vi "Fully Dynamic FPGA Interface Example.vi"() -> ()   [LabVIEW 2011]
uses:
  TypeDefs/Fully Dynamic FPGA Interface TypeDef.ctl
  <vilib>/Utility/sysdir.llb/System Directory Type.ctl
  <userlib>/_FPGA Interface Advanced Tools/FPGA Interface Base/FPGA Interface Base.lvclass
  <userlib>/_FPGA Interface Advanced Tools/FPGA Bitfile Utility/Get Register Map.vi
  <userlib>/_FPGA Interface Advanced Tools/FPGA Bitfile Utility/Get Base Address.vi
  <vilib>/rvi/Utilities/XML/nirviXML_GetValue.vi
  <vilib>/rvi/Utilities/XML/nirviXML_GetValue_String.vi
  <vilib>/rvi/Bitfile/niFpgaReadBitfileXml_VIRegisterMap.vi
  <vilib>/rvi/Utilities/XML/nirviXML_GetValue_U32.vi
  <vilib>/Utility/VariantDataType/GetTypeInfo.vi
  <vilib>/Utility/VariantDataType/GetArrayInfo.vi
  <userlib>/_FPGA Interface Advanced Tools/FPGA Interface Base/FPGA Read By Name - Boolean.vi
  <userlib>/_FPGA Interface Advanced Tools/FPGA Interface Base/FPGA Read By Name - I8.vi
  <userlib>/_FPGA Interface Advanced Tools/FPGA Interface Base/FPGA Read By Name - I16.vi
  <userlib>/_FPGA Interface Advanced Tools/FPGA Interface Base/FPGA Read By Name - I32.vi
  <userlib>/_FPGA Interface Advanced Tools/FPGA Interface Base/FPGA Read By Name - I64.vi
  <userlib>/_FPGA Interface Advanced Tools/FPGA Interface Base/FPGA Read By Name - U8.vi
  <userlib>/_FPGA Interface Advanced Tools/FPGA Interface Base/FPGA Read By Name - U16.vi
  <userlib>/_FPGA Interface Advanced Tools/FPGA Interface Base/FPGA Read By Name - U32.vi
  <userlib>/_FPGA Interface Advanced Tools/FPGA Interface Base/FPGA Read By Name - U64.vi
  <userlib>/_FPGA Interface Advanced Tools/FPGA Interface Base/FPGA Read Array By Name - Boolean.vi
  <userlib>/_FPGA Interface Advanced Tools/FPGA Interface Base/FPGA Read Array By Name - I8.vi
  <userlib>/_FPGA Interface Advanced Tools/FPGA Interface Base/FPGA Read Array By Name - I16.vi
  <userlib>/_FPGA Interface Advanced Tools/FPGA Interface Base/FPGA Read Array By Name - I32.vi
  <userlib>/_FPGA Interface Advanced Tools/FPGA Interface Base/FPGA Read Array By Name - I64.vi
  <userlib>/_FPGA Interface Advanced Tools/FPGA Interface Base/FPGA Read Array By Name - U8.vi
  <userlib>/_FPGA Interface Advanced Tools/FPGA Interface Base/FPGA Read Array By Name - U16.vi
  <userlib>/_FPGA Interface Advanced Tools/FPGA Interface Base/FPGA Read Array By Name - U32.vi
  <userlib>/_FPGA Interface Advanced Tools/FPGA Interface Base/FPGA Read Array By Name - U64.vi
  <userlib>/_FPGA Interface Advanced Tools/FPGA Interface Base/FPGA Write By Name - Boolean.vi
  <userlib>/_FPGA Interface Advanced Tools/FPGA Interface Base/FPGA Write By Name - I8.vi
  <userlib>/_FPGA Interface Advanced Tools/FPGA Interface Base/FPGA Write By Name - I16.vi
  <userlib>/_FPGA Interface Advanced Tools/FPGA Interface Base/FPGA Write By Name - I32.vi
  <userlib>/_FPGA Interface Advanced Tools/FPGA Interface Base/FPGA Write By Name - I64.vi
  <userlib>/_FPGA Interface Advanced Tools/FPGA Interface Base/FPGA Write By Name - U8.vi
  <userlib>/_FPGA Interface Advanced Tools/FPGA Interface Base/FPGA Write By Name - U16.vi
  <userlib>/_FPGA Interface Advanced Tools/FPGA Interface Base/FPGA Write By Name - U32.vi
  <userlib>/_FPGA Interface Advanced Tools/FPGA Interface Base/FPGA Write By Name - U64.vi
  <userlib>/_FPGA Interface Advanced Tools/FPGA Interface Base/FPGA Write Array By Name - Boolean.vi
  <userlib>/_FPGA Interface Advanced Tools/FPGA Interface Base/FPGA Write Array By Name - I8.vi
  <userlib>/_FPGA Interface Advanced Tools/FPGA Interface Base/FPGA Write Array By Name - I16.vi
  <userlib>/_FPGA Interface Advanced Tools/FPGA Interface Base/FPGA Write Array By Name - I32.vi
  <userlib>/_FPGA Interface Advanced Tools/FPGA Interface Base/FPGA Write Array By Name - I64.vi
  <userlib>/_FPGA Interface Advanced Tools/FPGA Interface Base/FPGA Write Array By Name - U8.vi
  <userlib>/_FPGA Interface Advanced Tools/FPGA Interface Base/FPGA Write Array By Name - U16.vi
  <userlib>/_FPGA Interface Advanced Tools/FPGA Interface Base/FPGA Write Array By Name - U32.vi
  <userlib>/_FPGA Interface Advanced Tools/FPGA Interface Base/FPGA Write Array By Name - U64.vi
  <userlib>/_FPGA Interface Advanced Tools/FPGA Bitfile Utility/FPGA Bitfile Utility.lvlib
panel:
  in  "RIO Resource":refnum<visa-resource-name>="RIO0"
  out "Boolean Array Read":bool[](array[boolean])
  in  "Boolean Array Write":bool[](array[boolean])
  in  "Numeric Array Write":dbl[](array[numeric])
  out "Numeric Array Read":dbl[](array[numeric])
  in  "Numeric Write":dbl
  out "Numeric Read":dbl
  in  "Boolean Write":bool
  out "Bool Read":bool
  in  "Write":bool
  in  "Read":bool
  in  "Multicolumn Listbox":i32(listbox)
  in  "Stop FPGA":bool
  in  "Run FPGA":bool
  in  "Select Bitfile":bool
  out "Bifile Path":path
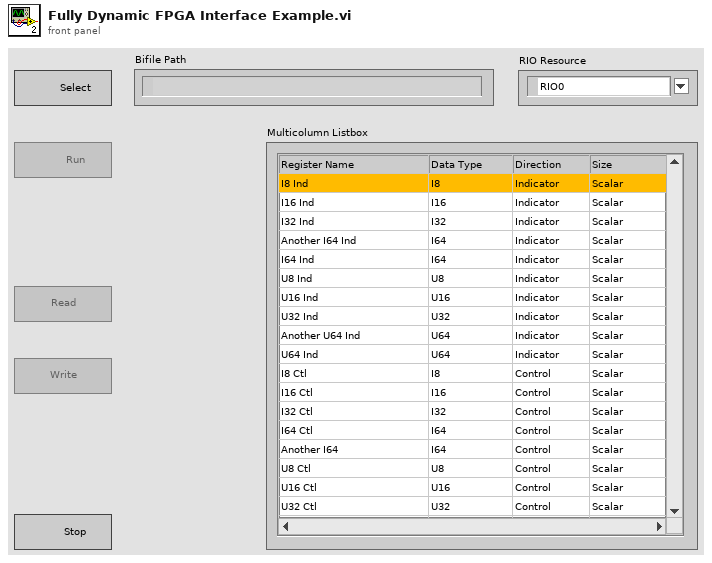
[diagram p1: front panel]
types:
  T1 = typedef "Fully Dynamic FPGA Interface TypeDef.ctl" = enum16{"Idle", "Init", "Read", "Write"}
  T2 = enum8{"Enabled", "Disabled", "Disabled and Grayed Out"}
  T3 = typedef "System Directory Type.ctl" = i32
  T4 = typedef "FPGA Bitfile Utility.lvlib/Control_Indicator Info.ctl" = cluster{"Array?":bool, "Data Type":T5, "Address":u32, "Num Elements":u32, "Name":string}
  T5 = typedef "niFpgaDataTypeControl.ctl" = enum32{"Boolean", "I8", "I16", "I32", "I64", "U8", "U16", "U32", "U64", "FXP", "CustomControl"}
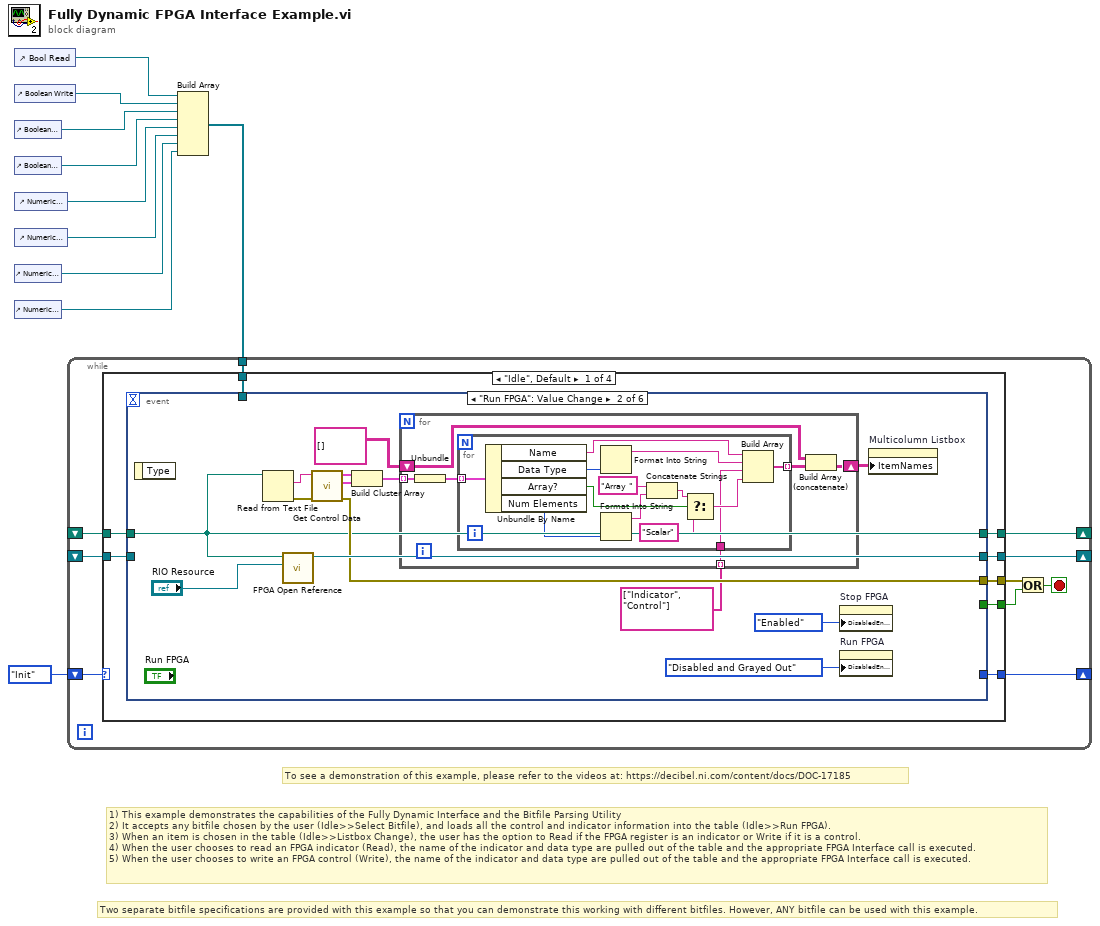
[diagram p0: block diagram]
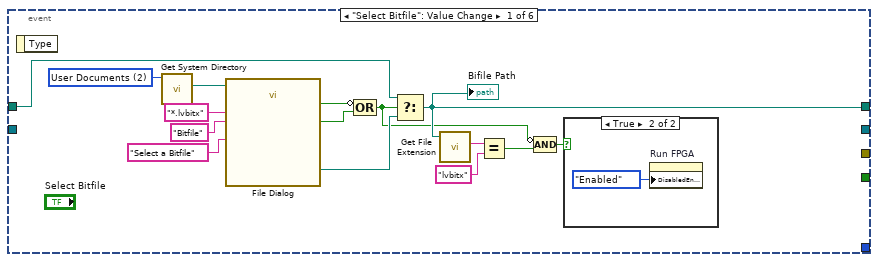
[diagram p2: hidden frame]
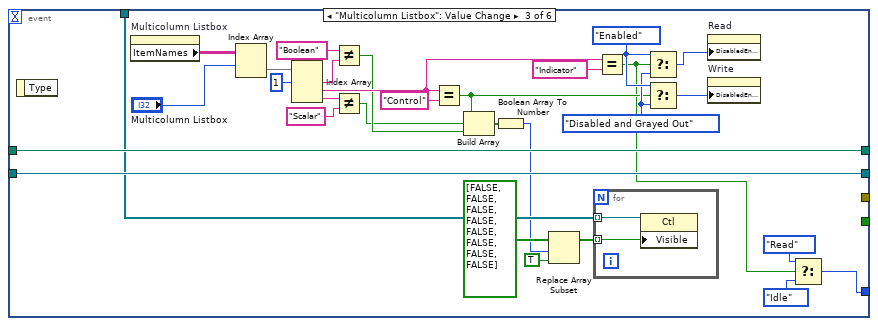
[diagram p4: hidden frame]
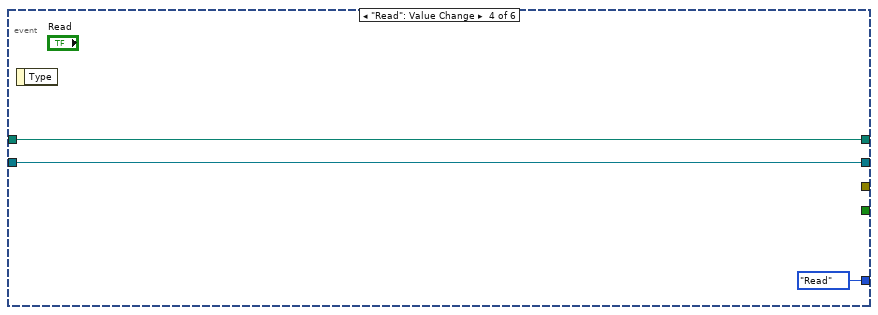
[diagram p5: hidden frame]
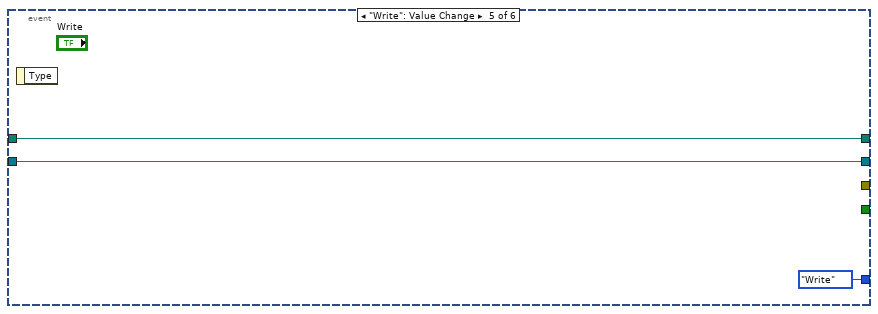
[diagram p6: hidden frame]
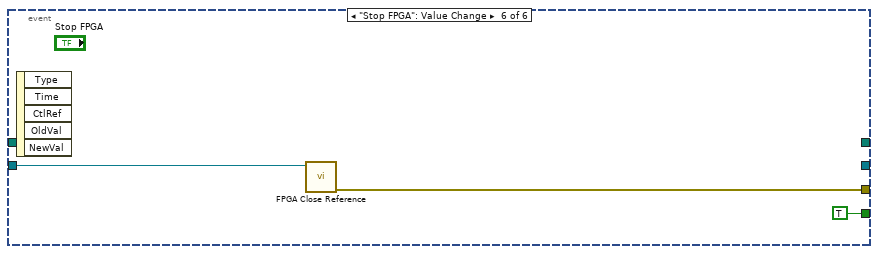
[diagram p7: hidden frame]
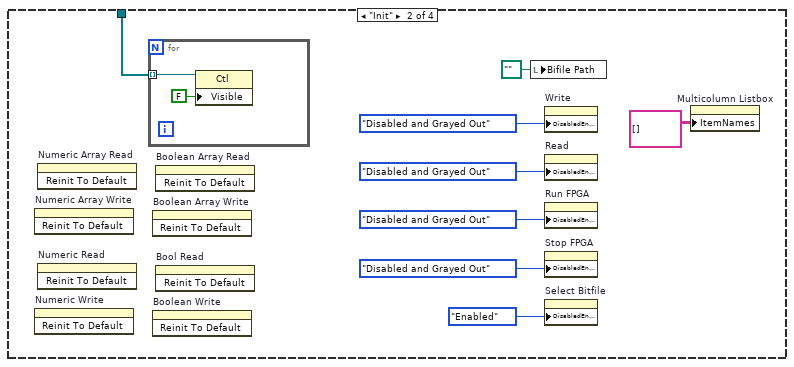
[diagram p8: hidden frame]
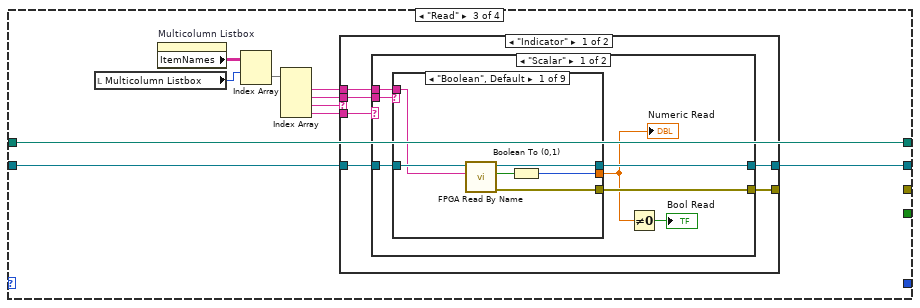
[diagram p9: hidden frame]
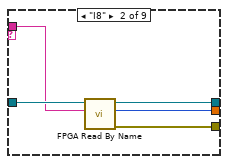
[diagram p10: hidden frame]
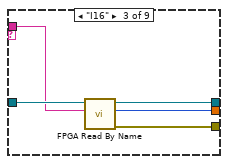
[diagram p11: hidden frame]
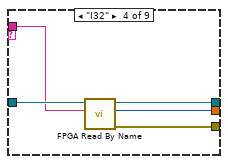
[diagram p12: hidden frame]
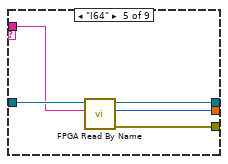
[diagram p13: hidden frame]
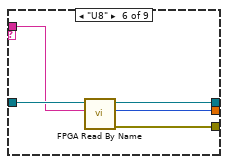
[diagram p14: hidden frame]
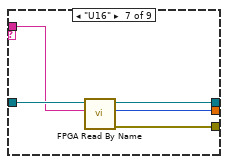
[diagram p15: hidden frame]
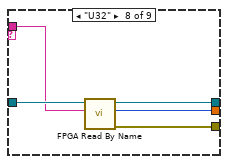
[diagram p16: hidden frame]
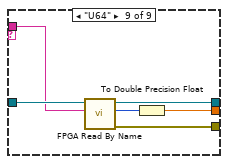
[diagram p17: hidden frame]
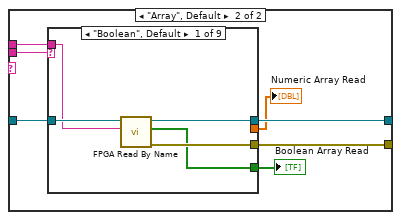
[diagram p18: hidden frame]
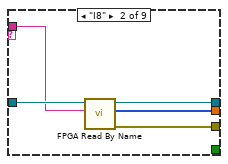
[diagram p19: hidden frame]
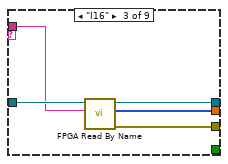
[diagram p20: hidden frame]
diagram:
  # "Two separate bitfile specifications are provided with this example so that you can demonstrate this working with different bitfiles. However, ANY bitfile can be used with this example."
  # "1) This example demonstrates the capabilities of the Fully Dynamic Interface and the Bitfile Parsing Utility\n2) It accepts any bitfile chosen by the user (Idle>>Select Bitfile), and loads all the control and indicator information into the table (Idle>>Run FPGA).\n3) When an item is chosen in the table (Idle>>Listbox Change), the user has the option to Read if the FPGA register is an indicator or Write if it is a control.\n4) When the user chooses to read an FPGA indicator (Read), the name of the indicator and data type are pulled out of the table and the appropriate FPGA Interface call is executed.\n5) When the user chooses to write an FPGA control (Write), the name of the indicator and data type are pulled out of the table and the appropriate FPGA Interface call is executed."
  # "To see a demonstration of this example, please refer to the videos at: https://decibel.ni.com/content/docs/DOC-17185"
  n1 = control-ref of="Bool Read"() -> (w10:refnum<vi>)
  n2 = control-ref of="Boolean Write"() -> (w6:refnum<vi>)
  n3 = control-ref of="Boolean Array Read"() -> (w7:refnum<vi>)
  n4 = control-ref of="Boolean Array Write"() -> (w8:refnum<vi>)
  n5 = control-ref of="Numeric Read"() -> (w5:refnum<vi>)
  n6 = control-ref of="Numeric Write"() -> (w4:refnum<vi>)
  n7 = control-ref of="Numeric Array Read"() -> (w3:refnum<vi>)
  n8 = control-ref of="Numeric Array Write"() -> (w2:refnum<vi>)
  n9 = Build Array(w10, w6, w7, w8, w5, w4, w3, w2) -> (w9:refnum<vi>[])
  n10 = while {
    shift-right: [w20] -> _
    shift-left: _ -> [w19]
    shift-right: [w18] -> _
    shift-left: _ -> [w17]
    tunnel: w9 -> [w13]
    shift-right: [w11] -> _
    shift-left: Fully_Dynamic_FPGA_Interface_TypeDef."Init" -> [w12]
    stop <- w15 stop-if-true
    n11 = case shown="\"Idle\", Default" w12 {
      tunnel: [w28 _ w129 w253] -> w20
      tunnel: w19 -> [w27 _ w129 w253]
      tunnel: [w26 _ w130 w254] -> w18
      tunnel: w17 -> [w25 _ w131 w255]
      tunnel: [w24 _ _ _] -> w16
      tunnel: [w23 _ _ _] -> w14
      tunnel: w13 -> [w22 w119 _ _]
      tunnel: [w21 _ _ _] -> w11
      frame "Idle", Default {
        n12 = event shown="[1] \"Run FPGA\": Value Change" {
          selector: _ -> [_ _ _ _ _ _]
          dyn-events: _ -> [_ _ _ _ _ _]
          timeout: _ -> [_ _ _ _ _ _]
          tunnel: [w34 w54 w98 w111 w113 _] -> w28
          tunnel: w27 -> [w35 w54 w98 w111 w113 _]
          tunnel: [_ w58 w99 w110 w114 _] -> w26
          tunnel: w25 -> [_ _ w99 w110 w114 w118]
          tunnel: [_ w55 _ _ _ w117] -> w24
          tunnel: [_ _ _ _ _ TRUE] -> w23
          tunnel: w22 -> [_ _ w95 _ _ _]
          tunnel: [_ _ w80 Fully_Dynamic_FPGA_Interface_TypeDef."Read" Fully_Dynamic_FPGA_Interface_TypeDef."Write" _] -> w21
          event "Select Bitfile": Value Change {
            w43 = T3 2 items=["User Home"=0, "User Desktop"=1, "User Documents"=2, "User Application Data"=3, "User Preferences"=4, "User Temporary"=5, "Public Documents"=6, "Public Application Data"=7, "Public Preferences"=8, "Public Cache"=13, "System Core Libraries"=9, "System Installed Libraries"=10, "Application Files"=11, "Boot Volume Root"=12] ("system directory type")
            n13 = event-data() -> ()  [unwired: 1 in, 1 out]
            n14 = call <vilib>:"Get System Directory.vi"("system directory type"=w43) -> ("system directory"=w42:path)  [unwired: 10 in]
            n15 = call "File Dialog"("start path"=w42, "prompt"="Select a Bitfile", "pattern (all files)"="*.lvbitx", "pattern label"="Bitfile") -> ("selected path"=w36:path, "exists"=w37:bool, "cancelled"=w38:bool)  [unwired: 8 in, 1 out]
            n16 = Compound Arithmetic op=OR(invert w37, w38) -> (w29:bool)
            n17 = Select(t=w35, s=w29, f=w36) -> (s? t:f=w34:path)
            "Bifile Path" <- w34
            n18 = call <vilib>:"Get File Extension.vi"("file"=w34) -> ("lowercase file extension"=w33:string)  [unwired: 7 in, 3 out]
            n19 = Equal?(x=w33, y="lvbitx") -> (x = y?=w31:bool)
            n20 = Compound Arithmetic op=AND(invert w29, w31) -> (w30:bool)
            n21 = case shown="True" w30 {
              frame False {
              }
              frame True {
                n22 = property on="Run FPGA" class="Bool"("DisabledEnum"=T2."Enabled" ("Disabled")) -> ()  [unwired: 2 in, 2 out]
              }
            }
          }
          event "Run FPGA": Value Change {
            n23 = event-data() -> ()  [unwired: 1 in, 1 out]
            n24 = Read from Text File(file (use dialog)=w54) -> (text=w57:string, error out=w56:errorcluster)  [unwired: 3 in, 2 out]
            n25 = call <userlib>:"FPGA Open Reference.vi"("FPGA Resource"="RIO Resource", "Bitfile Path"=w54) -> ("FPGA Session"=w58:refnum<class "FPGA Interface Base.lvclass">)  [unwired: 8 in, 1 out]
            n26 = call <userlib>:"Get Control Data.vi"("error in (no error)"=w56, "bitfile xml in"=w57) -> ("error out"=w55:errorcluster, "Controls"=w51:T4[], "Indicators"=w53:T4[])  [unwired: 6 in, 1 out]
            n27 = Build Cluster Array(w53, w51) -> (w52:cluster{"Controls":T4[]}[])
            n28 = for {
              tunnel: w52 -> [w64] mode=indexing
              tunnel: string[] ["Indicator", "Control"] -> [w63] mode=indexing
              shift-right: [w62] -> w49
              shift-left: string[][] [] -> [w61]
              n29 = Unbundle(w64) -> ("Controls"=w59:T4[])
              n30 = for {
                tunnel: w59 -> [w77] mode=indexing
                tunnel: [w66] -> w60 mode=indexing
                tunnel: w63 -> [w65]
                n31 = Unbundle By Name(w77) -> ("Name"=w69:string, "Data Type"=w76:T5, "Array?"=w75:bool, "Num Elements"=w74:u32)
                n32 = Format Into String(w76) -> (resulting string=w68:string)  [unwired: 3 in, 1 out]
                n33 = Format Into String(w74) -> (resulting string=w72:string)  [unwired: 3 in, 1 out]
                n34 = Concatenate Strings("Array " ("Name"), w72) -> (w71:string)
                n35 = Select(t=w71, s=w75, f="Scalar" ("Name")) -> (s? t:f=w67:string)
                n36 = Build Array(w69, w68, w65, w67) -> (w66:string[])
              }
              n37 = Build Array (concatenate)(w61, w60) -> (w62:string[][])
            }
            n38 = property on="Stop FPGA" class="Bool"("DisabledEnum"=T2."Enabled" ("Disabled")) -> ()  [unwired: 2 in, 2 out]
            n39 = property on="Run FPGA" class="Bool"("DisabledEnum"=T2."Disabled and Grayed Out" ("Disabled")) -> ()  [unwired: 2 in, 2 out]
            n40 = property on="Multicolumn Listbox" class="MCListbox (strict)"("ItemNames"=w49) -> ()  [unwired: 2 in, 2 out]
          }
          event "Multicolumn Listbox": Value Change {
            w97 = T2."Disabled and Grayed Out" ("Disabled")
            w102 = T2."Enabled" ("Disabled")
            n41 = event-data() -> ()  [unwired: 1 in, 1 out]
            n42 = property on="Multicolumn Listbox" class="MCListbox (strict)"() -> ("ItemNames"=w107:string[][])  [unwired: 2 in, 2 out]
            n43 = Index Array(array=w107, index (row)="Multicolumn Listbox") -> (element=w103:string[])  [unwired: 1 in]
            n44 = Index Array(array=w103, index #1=1 ("index")) -> (element #1=w90:string, element #2=w91:string, element #3=w87:string)  [unwired: 2 in]
            n45 = Not Equal?(x="Boolean", y=w90) -> (x != y?=w88:bool)
            n46 = Not Equal?(x=w87, y="Scalar") -> (x != y?=w83:bool)
            n47 = Equal?(x=w91, y="Control") -> (x = y?=w79:bool)
            n48 = Build Array(w79, w83, w88) -> (w85:bool[])
            n49 = Boolean Array To Number(Boolean array=w85) -> (number=w84:u32)
            n50 = Replace Array Subset(array=bool[] [FALSE, FALSE, FALSE, FALSE, FALSE, FALSE, FALSE, FALSE], new element=TRUE ("new element/subarray"), index=w84) -> (w94:bool[])
            n51 = for {
              tunnel: w95 -> [w109] mode=indexing
              tunnel: w94 -> [w108] mode=indexing
              n52 = property class="Ctl"(reference=w109, "Visible"=w108) -> ()  [unwired: 1 in, 2 out]
            }
            n53 = Equal?(x=w91, y="Indicator") -> (x = y?=w78:bool)
            n54 = Select(t=w102, s=w78, f=w97) -> (s? t:f=w100:T2)
            n55 = Select(t=w102, s=w79, f=w97) -> (s? t:f=w101:T2)
            n56 = property on="Read" class="Bool"("DisabledEnum"=w100) -> ()  [unwired: 2 in, 2 out]
            n57 = property on="Write" class="Bool"("DisabledEnum"=w101) -> ()  [unwired: 2 in, 2 out]
            n58 = Select(t=Fully_Dynamic_FPGA_Interface_TypeDef."Read", s=w78, f=Fully_Dynamic_FPGA_Interface_TypeDef."Idle") -> (s? t:f=w80:T1)
          }
          event "Read": Value Change {
            n59 = event-data() -> ()  [unwired: 1 in, 1 out]
          }
          event "Write": Value Change {
            n60 = event-data() -> ()  [unwired: 1 in, 1 out]
          }
          event "Stop FPGA": Value Change {
            n61 = event-data() -> ()  [unwired: 1 in, 5 out]
            n62 = call-dynamic "FPGA Close Reference.vi"("FPGA Session In"=w118) -> ("error out"=w117:errorcluster)  [unwired: 10 in]
          }
        }
      }
      frame "Init" {
        n63 = invoke on="Numeric Array Write" class="Arr (strict)" method="Reinit To Default"() -> ()  [unwired: 3 in, 3 out]
        n64 = invoke on="Numeric Write" class="DigNum (strict)" method="Reinit To Default"() -> ()  [unwired: 3 in, 3 out]
        n65 = invoke on="Numeric Array Read" class="Arr (strict)" method="Reinit To Default"() -> ()  [unwired: 3 in, 3 out]
        n66 = invoke on="Numeric Read" class="DigNum (strict)" method="Reinit To Default"() -> ()  [unwired: 3 in, 3 out]
        n67 = for {
          tunnel: w119 -> [w128] mode=indexing
          n68 = property class="Ctl"(reference=w128, "Visible"=FALSE) -> ()  [unwired: 1 in, 2 out]
        }
        n69 = invoke on="Boolean Array Write" class="Arr (strict)" method="Reinit To Default"() -> ()  [unwired: 3 in, 3 out]
        n70 = invoke on="Boolean Write" class="Bool (strict)" method="Reinit To Default"() -> ()  [unwired: 3 in, 3 out]
        n71 = invoke on="Boolean Array Read" class="Arr (strict)" method="Reinit To Default"() -> ()  [unwired: 3 in, 3 out]
        n72 = invoke on="Bool Read" class="Bool (strict)" method="Reinit To Default"() -> ()  [unwired: 3 in, 3 out]
        n73 = local write "Bifile Path"(path "" ("Bifile Path")) -> ()
        n74 = property on="Write" class="Bool"("DisabledEnum"=T2."Disabled and Grayed Out" ("Disabled")) -> ()  [unwired: 2 in, 2 out]
        n75 = property on="Read" class="Bool"("DisabledEnum"=T2."Disabled and Grayed Out" ("Disabled")) -> ()  [unwired: 2 in, 2 out]
        n76 = property on="Run FPGA" class="Bool"("DisabledEnum"=T2."Disabled and Grayed Out" ("Disabled")) -> ()  [unwired: 2 in, 2 out]
        n77 = property on="Stop FPGA" class="Bool"("DisabledEnum"=T2."Disabled and Grayed Out" ("Disabled")) -> ()  [unwired: 2 in, 2 out]
        n78 = property on="Select Bitfile" class="Bool"("DisabledEnum"=T2."Enabled" ("Disabled")) -> ()  [unwired: 2 in, 2 out]
        n79 = property on="Multicolumn Listbox" class="MCListbox (strict)"("ItemNames"=string[][] [] ("Item Names")) -> ()  [unwired: 2 in, 2 out]
      }
      frame "Read" {
        n80 = local read "Multicolumn Listbox"() -> (w137:i32)
        n81 = property on="Multicolumn Listbox" class="MCListbox (strict)"() -> ("ItemNames"=w138:string[][])  [unwired: 2 in, 2 out]
        n82 = Index Array(array=w138, index (row)=w137) -> (element=w136:string[])  [unwired: 1 in]
        n83 = Index Array(array=w136) -> (element #1=w134:string, element #2=w133:string, element #3=w135:string, element #4=w132:string)  [unwired: 4 in]
        n84 = case shown="\"Indicator\"" w135 {
          tunnel: w134 -> [w141 _]
          tunnel: w133 -> [w143 _]
          tunnel: w132 -> [w144 _]
          tunnel: w131 -> [w142 w252]
          tunnel: [w140 w252] -> w130
          tunnel: [w139 _] -> _
          frame "Indicator" {
            n85 = case shown="\"Scalar\"" w144 {
              tunnel: w143 -> [w151 w204]
              tunnel: w142 -> [w150 w203]
              tunnel: w141 -> [w149 w205]
              tunnel: [w148 w202] -> w140
              tunnel: [w147 w201] -> w139
              frame "Scalar" {
                n86 = case shown="\"Boolean\", Default" w151 {
                  tunnel: w150 -> [w157 w162 w167 w172 w177 w182 w187 w192 w198]
                  tunnel: w149 -> [w156 w161 w166 w171 w176 w181 w186 w191 w197]
                  tunnel: [w154 w160 w165 w170 w175 w180 w185 w190 w196] -> w148
                  tunnel: [w155 w159 w164 w169 w174 w179 w184 w189 w195] -> w147
                  tunnel: [w152 w158 w163 w168 w173 w178 w183 w188 w193] -> w145
                  frame "Boolean", Default {
                    n87 = call-poly <userlib>:"FPGA Read By Name.vi"("Indicator"=w156, "FPGA Session In"=w157) -> ("error out"=w155:errorcluster, "Value"=w153:bool, "FPGA Session Out"=w154:refnum<class "FPGA Interface Base.lvclass">)  [unwired: 7 in]
                    n88 = Boolean To (0,1)(Boolean=w153) -> (0, 1=w152:i16)
                  }
                  frame "I8" {
                    n89 = call-poly <userlib>:"FPGA Read By Name.vi"("Indicator"=w161, "FPGA Session In"=w162) -> ("error out"=w159:errorcluster, "Value"=w158:i8, "FPGA Session Out"=w160:refnum<class "FPGA Interface Base.lvclass">)  [unwired: 7 in]
                  }
                  frame "I16" {
                    n90 = call-poly <userlib>:"FPGA Read By Name.vi"("Indicator"=w166, "FPGA Session In"=w167) -> ("error out"=w164:errorcluster, "Value"=w163:i16, "FPGA Session Out"=w165:refnum<class "FPGA Interface Base.lvclass">)  [unwired: 7 in]
                  }
                  frame "I32" {
                    n91 = call-poly <userlib>:"FPGA Read By Name.vi"("Indicator"=w171, "FPGA Session In"=w172) -> ("error out"=w169:errorcluster, "Value"=w168:i32, "FPGA Session Out"=w170:refnum<class "FPGA Interface Base.lvclass">)  [unwired: 7 in]
                  }
                  frame "I64" {
                    n92 = call-poly <userlib>:"FPGA Read By Name.vi"("Indicator"=w176, "FPGA Session In"=w177) -> ("error out"=w174:errorcluster, "Value"=w173:i64, "FPGA Session Out"=w175:refnum<class "FPGA Interface Base.lvclass">)  [unwired: 7 in]
                  }
                  frame "U8" {
                    n93 = call-poly <userlib>:"FPGA Read By Name.vi"("Indicator"=w181, "FPGA Session In"=w182) -> ("error out"=w179:errorcluster, "Value"=w178:u8, "FPGA Session Out"=w180:refnum<class "FPGA Interface Base.lvclass">)  [unwired: 7 in]
                  }
                  frame "U16" {
                    n94 = call-poly <userlib>:"FPGA Read By Name.vi"("Indicator"=w186, "FPGA Session In"=w187) -> ("error out"=w184:errorcluster, "Value"=w183:u16, "FPGA Session Out"=w185:refnum<class "FPGA Interface Base.lvclass">)  [unwired: 7 in]
                  }
                  frame "U32" {
                    n95 = call-poly <userlib>:"FPGA Read By Name.vi"("Indicator"=w191, "FPGA Session In"=w192) -> ("error out"=w189:errorcluster, "Value"=w188:u32, "FPGA Session Out"=w190:refnum<class "FPGA Interface Base.lvclass">)  [unwired: 7 in]
                  }
                  frame "U64" {
                    n96 = call-poly <userlib>:"FPGA Read By Name.vi"("Indicator"=w197, "FPGA Session In"=w198) -> ("error out"=w195:errorcluster, "Value"=w194:u64, "FPGA Session Out"=w196:refnum<class "FPGA Interface Base.lvclass">)  [unwired: 7 in]
                    n97 = To Double Precision Float(number=w194) -> (double precision float=w193:dbl)
                  }
                }
                "Numeric Read" <- w145
                n98 = Not Equal To 0?(x=w145) -> (x != 0?=→"Bool Read":bool)
              }
              frame "Array", Default {
                n99 = case shown="\"Boolean\", Default" w204 {
                  tunnel: w203 -> [w210 w215 w220 w225 w230 w235 w240 w245 w251]
                  tunnel: w205 -> [w209 w214 w219 w224 w229 w234 w239 w244 w250]
                  tunnel: [w207 w213 w218 w223 w228 w233 w238 w243 w249] -> w202
                  tunnel: [w208 w212 w217 w222 w227 w232 w237 w242 w248] -> w201
                  tunnel: [_ w211 w216 w221 w226 w231 w236 w241 w246] -> w199
                  tunnel: [w206 _ _ _ _ _ _ _ _] -> w200
                  frame "Boolean", Default {
                    n100 = call-poly <userlib>:"FPGA Read By Name.vi"("Indicator"=w209, "FPGA Session In"=w210) -> ("error out"=w208:errorcluster, "Array"=w206:bool[], "FPGA Session Out"=w207:refnum<class "FPGA Interface Base.lvclass">)  [unwired: 7 in]
                  }
                  frame "I8" {
                    n101 = call-poly <userlib>:"FPGA Read By Name.vi"("Indicator"=w214, "FPGA Session In"=w215) -> ("error out"=w212:errorcluster, "Array"=w211:i8[], "FPGA Session Out"=w213:refnum<class "FPGA Interface Base.lvclass">)  [unwired: 7 in]
                  }
                  frame "I16" {
                    n102 = call-poly <userlib>:"FPGA Read By Name.vi"("Indicator"=w219, "FPGA Session In"=w220) -> ("error out"=w217:errorcluster, "Array"=w216:i16[], "FPGA Session Out"=w218:refnum<class "FPGA Interface Base.lvclass">)  [unwired: 7 in]
                  }
                  frame "I32" {
                    n103 = call-poly <userlib>:"FPGA Read By Name.vi"("Indicator"=w224, "FPGA Session In"=w225) -> ("error out"=w222:errorcluster, "Array"=w221:i32[], "FPGA Session Out"=w223:refnum<class "FPGA Interface Base.lvclass">)  [unwired: 7 in]
                  }
                  frame "I64" {
                    n104 = call-poly <userlib>:"FPGA Read By Name.vi"("Indicator"=w229, "FPGA Session In"=w230) -> ("error out"=w227:errorcluster, "Array"=w226:i64[], "FPGA Session Out"=w228:refnum<class "FPGA Interface Base.lvclass">)  [unwired: 7 in]
                  }
                  frame "U8" {
                    n105 = call-poly <userlib>:"FPGA Read By Name.vi"("Indicator"=w234, "FPGA Session In"=w235) -> ("error out"=w232:errorcluster, "Array"=w231:u8[], "FPGA Session Out"=w233:refnum<class "FPGA Interface Base.lvclass">)  [unwired: 7 in]
                  }
                  frame "U16" {
                    n106 = call-poly <userlib>:"FPGA Read By Name.vi"("Indicator"=w239, "FPGA Session In"=w240) -> ("error out"=w237:errorcluster, "Array"=w236:u16[], "FPGA Session Out"=w238:refnum<class "FPGA Interface Base.lvclass">)  [unwired: 7 in]
                  }
                  frame "U32" {
                    n107 = call-poly <userlib>:"FPGA Read By Name.vi"("Indicator"=w244, "FPGA Session In"=w245) -> ("error out"=w242:errorcluster, "Array"=w241:u32[], "FPGA Session Out"=w243:refnum<class "FPGA Interface Base.lvclass">)  [unwired: 7 in]
                  }
                  frame "U64" {
                    n108 = call-poly <userlib>:"FPGA Read By Name.vi"("Indicator"=w250, "FPGA Session In"=w251) -> ("error out"=w248:errorcluster, "Array"=w247:u64[], "FPGA Session Out"=w249:refnum<class "FPGA Interface Base.lvclass">)  [unwired: 7 in]
                    n109 = To Double Precision Float(number=w247) -> (double precision float=w246:dbl[])
                  }
                }
                "Boolean Array Read" <- w200
                "Numeric Array Read" <- w199
              }
            }
          }
          frame "Control", Default {
          }
        }
      }
      frame "Write" {
        n110 = local read "Multicolumn Listbox"() -> (w261:i32)
        n111 = property on="Multicolumn Listbox" class="MCListbox (strict)"() -> ("ItemNames"=w262:string[][])  [unwired: 2 in, 2 out]
        n112 = Index Array(array=w262, index (row)=w261) -> (element=w260:string[])  [unwired: 1 in]
        n113 = Index Array(array=w260) -> (element #1=w258:string, element #2=w257:string, element #3=w259:string, element #4=w256:string)  [unwired: 4 in]
        n114 = case shown="\"Control\"" w259 {
          tunnel: w258 -> [w265 _]
          tunnel: w257 -> [w267 _]
          tunnel: w256 -> [w268 _]
          tunnel: w255 -> [w266 w373]
          tunnel: [w264 w373] -> w254
          tunnel: [w263 _] -> _
          frame "Control" {
            n115 = case shown="\"Array\", Default" w268 {
              tunnel: w267 -> [w275 w326]
              tunnel: w266 -> [w274 w325]
              tunnel: w265 -> [w273 w327]
              tunnel: [w272 w324] -> w264
              tunnel: [w271 w323] -> w263
              frame "Scalar" {
                n116 = case shown="\"Boolean\", Default" w275 {
                  tunnel: w274 -> [w280 w285 w290 w295 w300 w305 w310 w315 w320]
                  tunnel: w273 -> [w279 w284 w289 w294 w299 w304 w309 w314 w319]
                  tunnel: [w277 w282 w287 w292 w297 w302 w307 w312 w317] -> w272
                  tunnel: [w278 w283 w288 w293 w298 w303 w308 w313 w318] -> w271
                  tunnel: "Boolean Write" -> [w276 _ _ _ _ _ _ _ _]
                  tunnel: "Numeric Write" -> [_ w281 w286 w291 w296 w301 w306 w311 w316]
                  frame "Boolean", Default {
                    n117 = call-poly <userlib>:"FPGA Write By Name.vi"("Value"=w276, "Control"=w279, "FPGA Session In"=w280) -> ("error out"=w278:errorcluster, "FPGA Session Out"=w277:refnum<class "FPGA Interface Base.lvclass">)  [unwired: 7 in]
                  }
                  frame "I8" {
                    n118 = call-poly <userlib>:"FPGA Write By Name.vi"("Value"=w281, "Control"=w284, "FPGA Session In"=w285) -> ("error out"=w283:errorcluster, "FPGA Session Out"=w282:refnum<class "FPGA Interface Base.lvclass">)  [unwired: 7 in]
                  }
                  frame "I16" {
                    n119 = call-poly <userlib>:"FPGA Write By Name.vi"("Value"=w286, "Control"=w289, "FPGA Session In"=w290) -> ("error out"=w288:errorcluster, "FPGA Session Out"=w287:refnum<class "FPGA Interface Base.lvclass">)  [unwired: 7 in]
                  }
                  frame "I32" {
                    n120 = call-poly <userlib>:"FPGA Write By Name.vi"("Value"=w291, "Control"=w294, "FPGA Session In"=w295) -> ("error out"=w293:errorcluster, "FPGA Session Out"=w292:refnum<class "FPGA Interface Base.lvclass">)  [unwired: 7 in]
                  }
                  frame "I64" {
                    n121 = call-poly <userlib>:"FPGA Write By Name.vi"("Value"=w296, "Control"=w299, "FPGA Session In"=w300) -> ("error out"=w298:errorcluster, "FPGA Session Out"=w297:refnum<class "FPGA Interface Base.lvclass">)  [unwired: 7 in]
                  }
                  frame "U8" {
                    n122 = call-poly <userlib>:"FPGA Write By Name.vi"("Value"=w301, "Control"=w304, "FPGA Session In"=w305) -> ("error out"=w303:errorcluster, "FPGA Session Out"=w302:refnum<class "FPGA Interface Base.lvclass">)  [unwired: 7 in]
                  }
                  frame "U16" {
                    n123 = call-poly <userlib>:"FPGA Write By Name.vi"("Value"=w306, "Control"=w309, "FPGA Session In"=w310) -> ("error out"=w308:errorcluster, "FPGA Session Out"=w307:refnum<class "FPGA Interface Base.lvclass">)  [unwired: 7 in]
                  }
                  frame "U32" {
                    n124 = call-poly <userlib>:"FPGA Write By Name.vi"("Value"=w311, "Control"=w314, "FPGA Session In"=w315) -> ("error out"=w313:errorcluster, "FPGA Session Out"=w312:refnum<class "FPGA Interface Base.lvclass">)  [unwired: 7 in]
                  }
                  frame "U64" {
                    n125 = call-poly <userlib>:"FPGA Write By Name.vi"("Value"=w316, "Control"=w319, "FPGA Session In"=w320) -> ("error out"=w318:errorcluster, "FPGA Session Out"=w317:refnum<class "FPGA Interface Base.lvclass">)  [unwired: 7 in]
                  }
                }
              }
              frame "Array", Default {
                n126 = case shown="\"Boolean\", Default" w326 {
                  tunnel: w325 -> [w332 w337 w342 w347 w352 w357 w362 w367 w372]
                  tunnel: w327 -> [w331 w336 w341 w346 w351 w356 w361 w366 w371]
                  tunnel: [w329 w335 w340 w345 w350 w355 w360 w365 w370] -> w324
                  tunnel: [w330 w334 w339 w344 w349 w354 w359 w364 w369] -> w323
                  tunnel: "Numeric Array Write" -> [_ w333 w338 w343 w348 w353 w358 w363 w368]
                  tunnel: "Boolean Array Write" -> [w328 _ _ _ _ _ _ _ _]
                  frame "Boolean", Default {
                    n127 = call-poly <userlib>:"FPGA Write By Name.vi"("Array"=w328, "Control"=w331, "FPGA Session In"=w332) -> ("error out"=w330:errorcluster, "FPGA Session Out"=w329:refnum<class "FPGA Interface Base.lvclass">)  [unwired: 7 in]
                  }
                  frame "I8" {
                    n128 = call-poly <userlib>:"FPGA Write By Name.vi"("Array"=w333, "Control"=w336, "FPGA Session In"=w337) -> ("error out"=w334:errorcluster, "FPGA Session Out"=w335:refnum<class "FPGA Interface Base.lvclass">)  [unwired: 7 in]
                  }
                  frame "I16" {
                    n129 = call-poly <userlib>:"FPGA Write By Name.vi"("Array"=w338, "Control"=w341, "FPGA Session In"=w342) -> ("error out"=w339:errorcluster, "FPGA Session Out"=w340:refnum<class "FPGA Interface Base.lvclass">)  [unwired: 7 in]
                  }
                  frame "I32" {
                    n130 = call-poly <userlib>:"FPGA Write By Name.vi"("Array"=w343, "Control"=w346, "FPGA Session In"=w347) -> ("error out"=w344:errorcluster, "FPGA Session Out"=w345:refnum<class "FPGA Interface Base.lvclass">)  [unwired: 7 in]
                  }
                  frame "I64" {
                    n131 = call-poly <userlib>:"FPGA Write By Name.vi"("Array"=w348, "Control"=w351, "FPGA Session In"=w352) -> ("error out"=w349:errorcluster, "FPGA Session Out"=w350:refnum<class "FPGA Interface Base.lvclass">)  [unwired: 7 in]
                  }
                  frame "U8" {
                    n132 = call-poly <userlib>:"FPGA Write By Name.vi"("Array"=w353, "Control"=w356, "FPGA Session In"=w357) -> ("error out"=w354:errorcluster, "FPGA Session Out"=w355:refnum<class "FPGA Interface Base.lvclass">)  [unwired: 7 in]
                  }
                  frame "U16" {
                    n133 = call-poly <userlib>:"FPGA Write By Name.vi"("Array"=w358, "Control"=w361, "FPGA Session In"=w362) -> ("error out"=w359:errorcluster, "FPGA Session Out"=w360:refnum<class "FPGA Interface Base.lvclass">)  [unwired: 7 in]
                  }
                  frame "U32" {
                    n134 = call-poly <userlib>:"FPGA Write By Name.vi"("Array"=w363, "Control"=w366, "FPGA Session In"=w367) -> ("error out"=w364:errorcluster, "FPGA Session Out"=w365:refnum<class "FPGA Interface Base.lvclass">)  [unwired: 7 in]
                  }
                  frame "U64" {
                    n135 = call-poly <userlib>:"FPGA Write By Name.vi"("Array"=w368, "Control"=w371, "FPGA Session In"=w372) -> ("error out"=w369:errorcluster, "FPGA Session Out"=w370:refnum<class "FPGA Interface Base.lvclass">)  [unwired: 7 in]
                  }
                }
              }
            }
          }
          frame "Indicator", Default {
          }
        }
      }
    }
    n136 = Or(x=w16, y=w14) -> (x .or. y?=w15:bool)
  }
